vi "Read 1Pin 1Sampe Boolean.vi"(8 "error in (no error)":errorcluster, 10 "Pin":u8, 11 "MicroDAQ.lvlib:Digital Input.lvclass":refnum<class "Digital Input.lvclass">) -> (0 "error out":errorcluster, 2 "data":bool, 3 "MicroDAQ.lvlib:Digital Input.lvclass out":refnum<class "Digital Input.lvclass">)   [LabVIEW 2009, in "MicroDAQ.lvlib" / "Digital Input.lvclass"]
doc: "Reads a single Boolean sample from digital input channel composed of a single line."
uses:
  <instrlib>/MicroDAQ/Channel/Digital Input/Digital Input.lvclass
  <instrlib>/MicroDAQ/Mlink library wraper/mlink.lvlib
  <instrlib>/MicroDAQ/Channel/Channel.lvclass
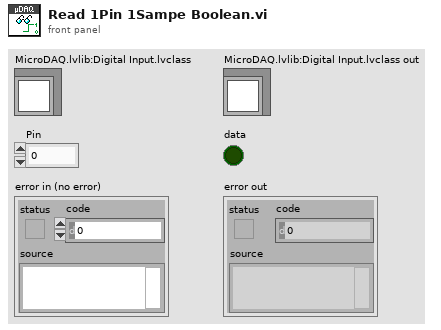
[diagram p1: front panel]
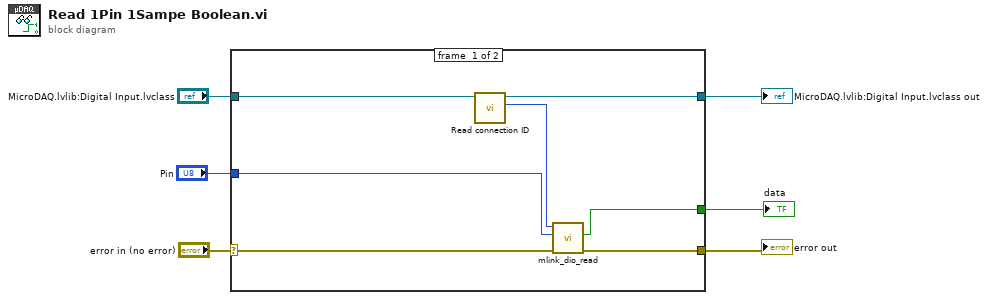
[diagram p0: block diagram]
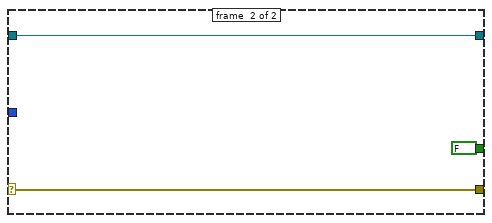
[diagram p2: hidden frame]
diagram:
  n1 = case shown="No Error" "error in (no error)" {
    selector: "error in (no error)" -> [w7 w14]
    tunnel: [w13 w14] -> w5
    tunnel: "MicroDAQ.lvlib:Digital Input.lvclass" -> [w9 w16]
    tunnel: [w12 w16] -> w3
    tunnel: "Pin" -> [w8 _]
    tunnel: [w10 FALSE ("state")] -> w1
    frame #0 {
      n2 = call <instrlib>:"Read connection ID.vi"("Task in"=w9) -> ("connection ID"=w11:i32, "Task out"=w12:refnum<class "Digital Input.lvclass">)  [unwired: 9 in]
      n3 = call <instrlib>:"mlink_dio_read.vi"("error in (no error)"=w7, "pin"=w8, "connection ID"=w11) -> ("error out"=w13:errorcluster, "state"=w10:bool)  [unwired: 6 in, 1 out]
    }
    frame #1 {
    }
  }
  "error out" <- w5
  "MicroDAQ.lvlib:Digital Input.lvclass out" <- w3
  "data" <- w1
